vi "Analyze Data.vi"(0 "Données météo":dynamicdata(waveform), 11 "entrée d'erreur":errorcluster) -> (4 "Temps":dbl, 6 "Température":dbl, 8 "Vitesse du vent":dbl, 15 "sortie d'erreur":errorcluster)   [LabVIEW 2009]
uses:
  Instance           2 20Saved   Analyze Data .vi
  Instance           5 20Saved   Analyze Data .vi
  Instance           4 20Saved   Analyze Data .vi
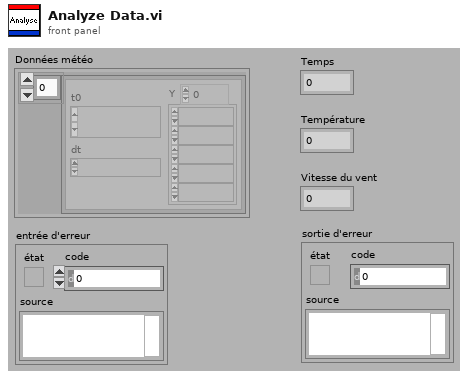
[diagram p1: front panel]
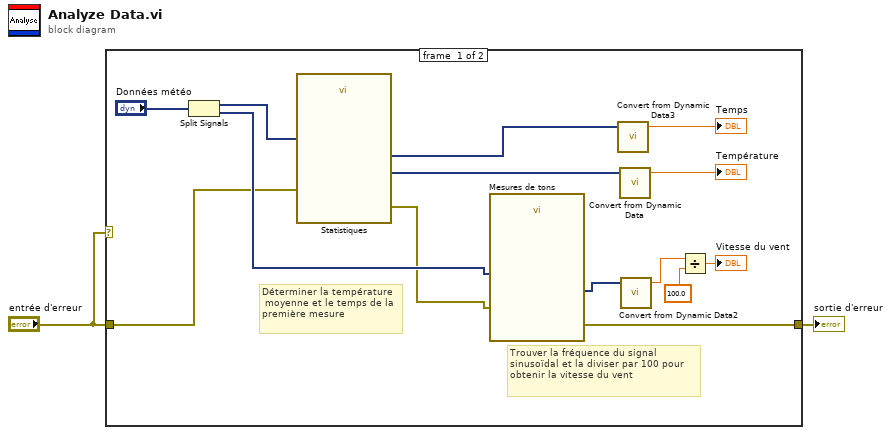
[diagram p0: block diagram]
diagram:
  n1 = case "Structure Condition" shown="Pas d'erreur" "entrée d'erreur" {
    tunnel: "entrée d'erreur" -> [w3 w17]
    tunnel: [w9 w17] -> w2
    frame #0 {
      # "Trouver la fréquence du signal sinusoïdal et la diviser par 100 pour obtenir la vitesse du vent"
      # "Déterminer la température\n moyenne et le temps de la première mesure"
      n2 = Split Signals ("Désassembler des signaux")("Données météo") -> (w7:dynamicdata, w10:dynamicdata)  [unwired: 2 in]
      n3 = call "Statistiques"("Signals"=w7, "error in (no error)"=w3) -> ("Arithmetic Mean"=w5:dynamicdata, "First Time"=w6:dynamicdata, "error out"=w4:errorcluster)  [unwired: 23 in]
      n4 = call "Mesures de tons"("error in (no error)"=w4, "Signals"=w10) -> ("error out"=w9:errorcluster, "Frequency"=w8:dynamicdata)  [unwired: 8 in]
      n5 = call "Convert from Dynamic Data3"("Dynamic Data Type"=w6) -> ("Scalar"=→"Temps":dbl)  [unwired: 3 in]
      n6 = call "Convert from Dynamic Data"("Dynamic Data Type"=w5) -> ("Scalar"=→"Température":dbl)  [unwired: 3 in]
      n7 = call "Convert from Dynamic Data2"("Dynamic Data Type"=w8) -> ("Scalar"=w12:dbl)  [unwired: 3 in]
      n8 = Divide ("Diviser")(x=w12, y=100.0) -> (x/y=→"Vitesse du vent":dbl)
    }
    frame #1 {
    }
  }
  "sortie d'erreur" <- w2
